vi "Autonomous Independent.vi"() -> ()   [LabVIEW 2019]
doc: "This VI is called when autonomous begins, and will automatically be terminated when autonomous ends. You can carry out timed or sensor driven robot movement independently without needing to return to the caller."
uses:
  <vilib>/Rock Robotics/WPI/Solenoid/WPI_SolenoidValue.ctl
  <vilib>/Rock Robotics/WPI/Utilities/WPI_GetSetVariantRefNum.vi
  <vilib>/Rock Robotics/Network Tables/NT Read String.vi
  <vilib>/Rock Robotics/Network Tables/NT Write Numeric Array.vi
  <vilib>/Rock Robotics/WPI/RobotDrive/WPI_RobotDriveArcadeDrive_Standard(NoSaturation).vi
  <vilib>/Rock Robotics/WPI/Solenoid/WPI_SolenoidSetEnum.vi
panel:
  in  "Polycord 3":dbl=-0.8 format="%#_13g"
  in  "Polycord 2":dbl=-0.8 format="%#_13g"
  in  "Angle 2":dbl
  in  "Speed 2":dbl
  in  "radius 2":dbl=20.0
  in  "angle 2":dbl=100.0
  in  "Inches Forward 2":dbl=26.0
  in  "Angle":dbl
  in  "Speed":dbl
  in  "radius":dbl=20.0
  in  "angle":dbl=100.0
  in  "Inches Forward":dbl=26.0
  # "Be sure to right-click and choose Data Operations>>Make Current Value default if you want to save the array values with the VI"
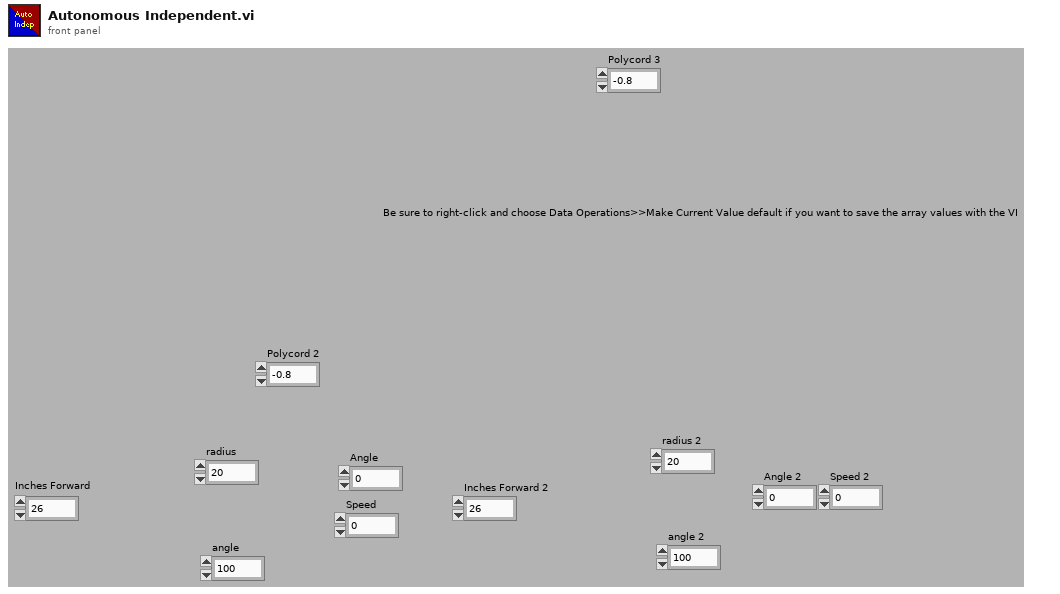
[diagram p1: front panel]
types:
  T1 = typedef "WPI_JoystickDevRef.ctl" = cluster{"Device":T2}
  T2 = typedef "WPI_JoystickDeviceEnum.ctl" = enum16{"USB 0", "USB 1", "USB 2", "USB 3", "USB 4", "USB 5"}
  T3 = typedef "WPI_SolenoidValue.ctl" = enum16{"Off", "On", "Forward", "Reverse"}
  T4 = typedef "WPI_RobotDriveDevRef.ctl" = cluster{"DevStatus":errorcluster, "Motors[]":T5[], "Square Inputs":bool, "Max Output":dbl}
  T5 = typedef "WPI_MotorControlDeviceRef.ctl" = cluster{"DeviceStatus":errorcluster, "Type":T6, "PWM":cluster{"PWM Channel":T7, "DeadBand":T8}, "CAN":cluster{"Device Number":u8, "SetOutput VI Ref":variant, "GetOutput VI Ref":variant, "Enable VI Ref":variant, "Disable VI Ref":variant, "Data":variant}, "Invert":bool, "DIO PWM":cluster{"PWM \"Enable\" Channel":T7, "DIOChannel":T9, "PWM Rate":dbl}}
  T6 = typedef "WPI_MotorControlType.ctl" = enum16{"PWM", "CAN", "DIO PWM"}
  T7 = typedef "FPGA_DIOPWMChannel.ctl" = enum8{"PWM 0", "PWM 1", "PWM 2", "PWM 3", "PWM 4", "PWM 5", "PWM 6", "PWM 7", "PWM 8", "PWM 9", "PWM MXP 0", "PWM MXP 1", "PWM MXP 2", "PWM MXP 3", "PWM MXP 4", "PWM MXP 5", "PWM MXP 6", "PWM MXP 7", "PWM MXP 8", "PWM MXP 9", "Invalid"}
  T8 = typedef "WPI_PWMDeadband.ctl" = cluster{"Name":string, "maxPositivePwm":i32, "minPositivePwm":i32, "centerPwm":i32, "maxNegativePwm":i32, "minNegativePwm":i32, "angularRange":u16}
  T9 = typedef "FPGA_DIOChannel.ctl" = enum8{"DIO 0", "DIO 1", "DIO 2", "DIO 3", "DIO 4", "DIO 5", "DIO 6", "DIO 7", "DIO 8", "DIO 9", "DIO MXP 0", "DIO MXP 1", "DIO MXP 2", "DIO MXP 3", "DIO MXP 4", "DIO MXP 5", "DIO MXP 6", "DIO MXP 7", "DIO MXP 8", "DIO MXP 9", "DIO MXP 10", "DIO MXP 11", "DIO MXP 12", "DIO MXP 13", "DIO MXP 14", "DIO MXP 15", "SPI Port CS1", "SPI Port CS2", "SPI Port CS3", "SPI Port MISO", "SPI Port MOSI", "Invalid"}
  T10 = typedef "WPI_SolenoidDevRef.ctl" = cluster{"DevStatus":errorcluster, "Pneumatics Control Module":u8, "Forward Solenoid Channel":T11, "Reverse Solenoid Channel":T11}
  T11 = typedef "WPI_SolenoidChannel.ctl" = enum8{"Solenoid 0", "Solenoid 1", "Solenoid 2", "Solenoid 3", "Solenoid 4", "Solenoid 5", "Solenoid 6", "Solenoid 7", "Invalid"}
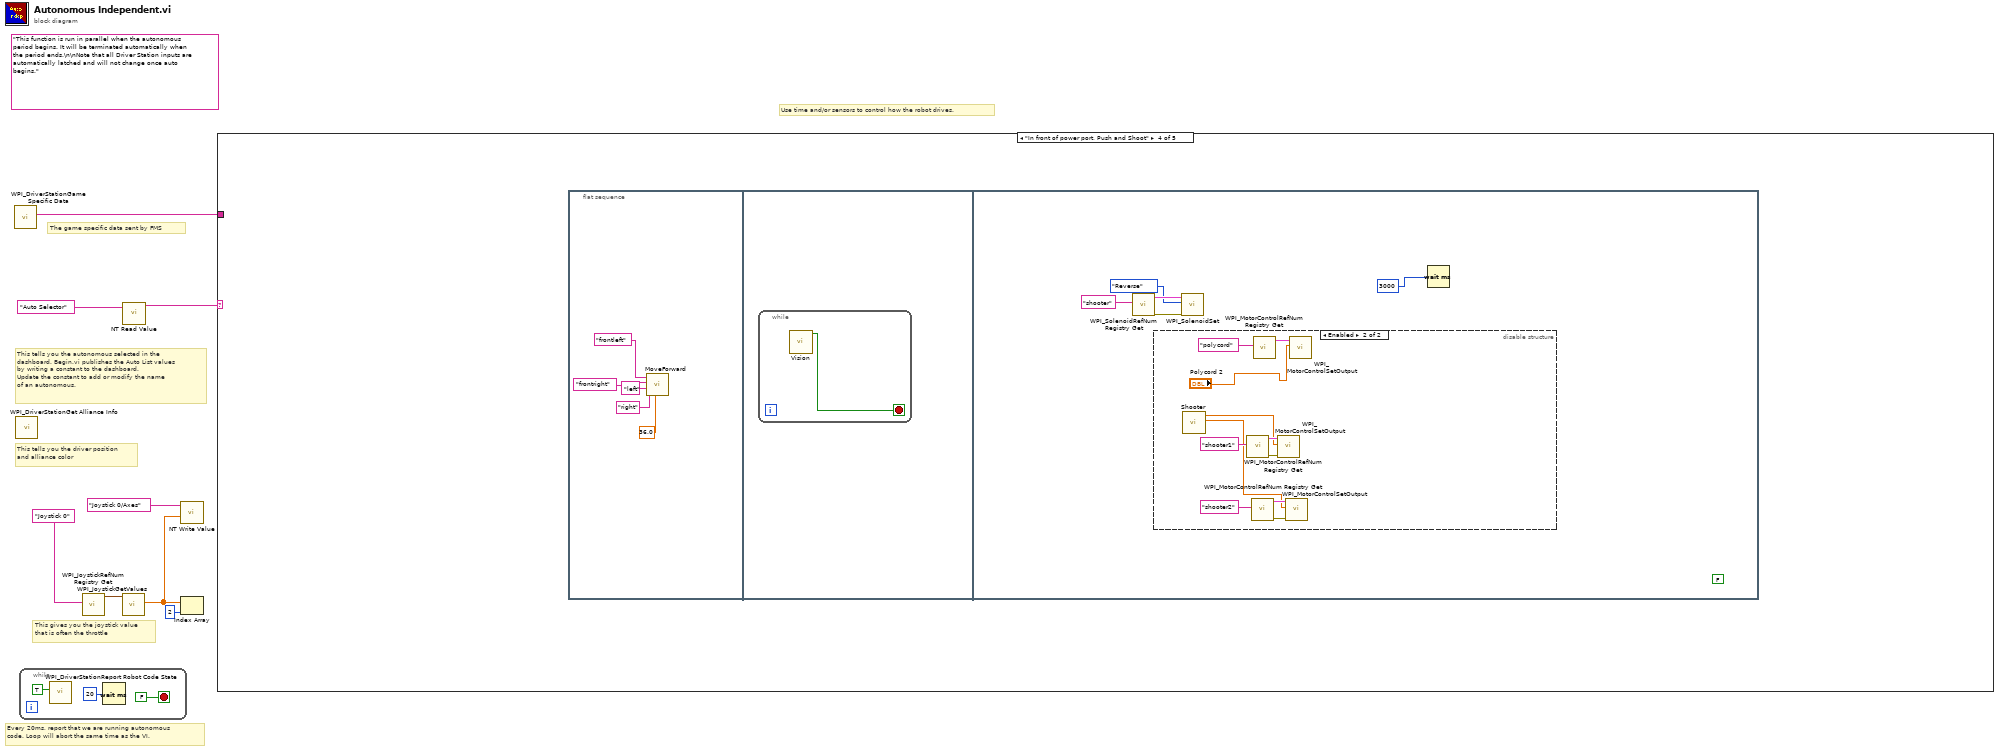
[diagram p0: block diagram]
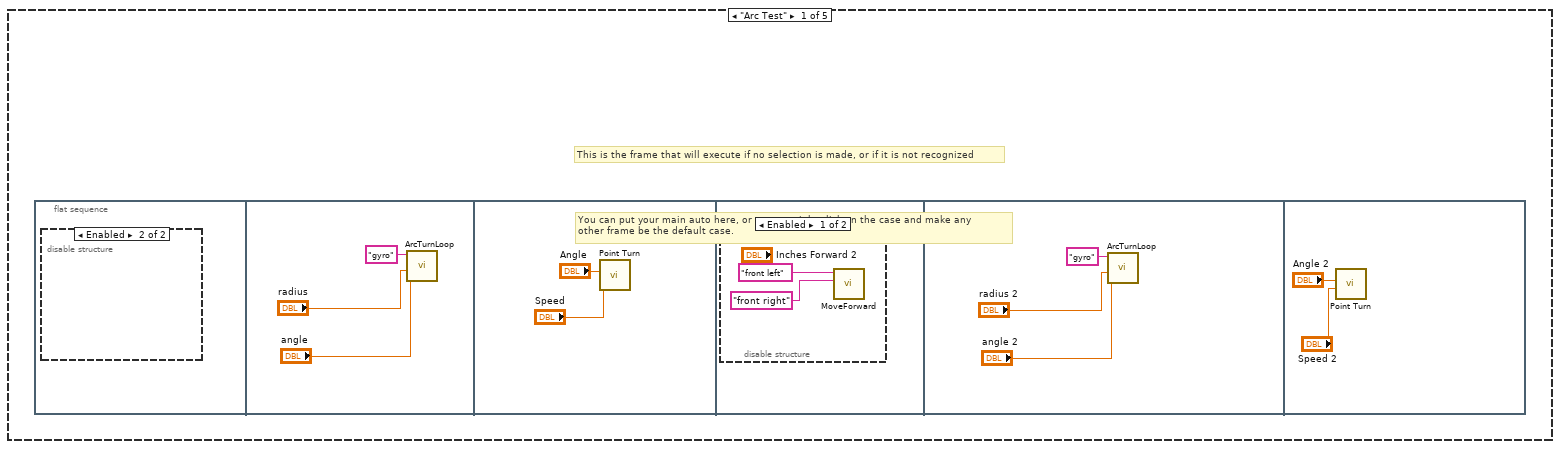
[diagram p2: hidden frame]
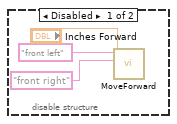
[diagram p3: hidden frame]
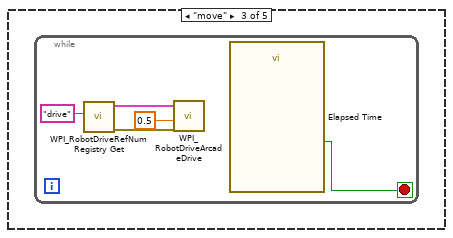
[diagram p6: hidden frame]
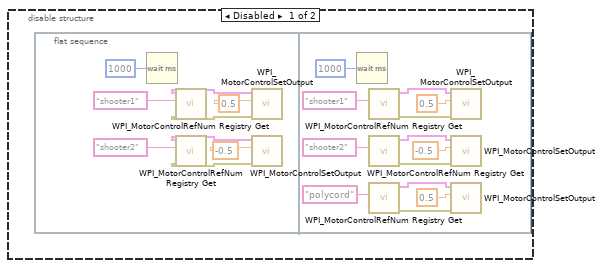
[diagram p7: hidden frame]
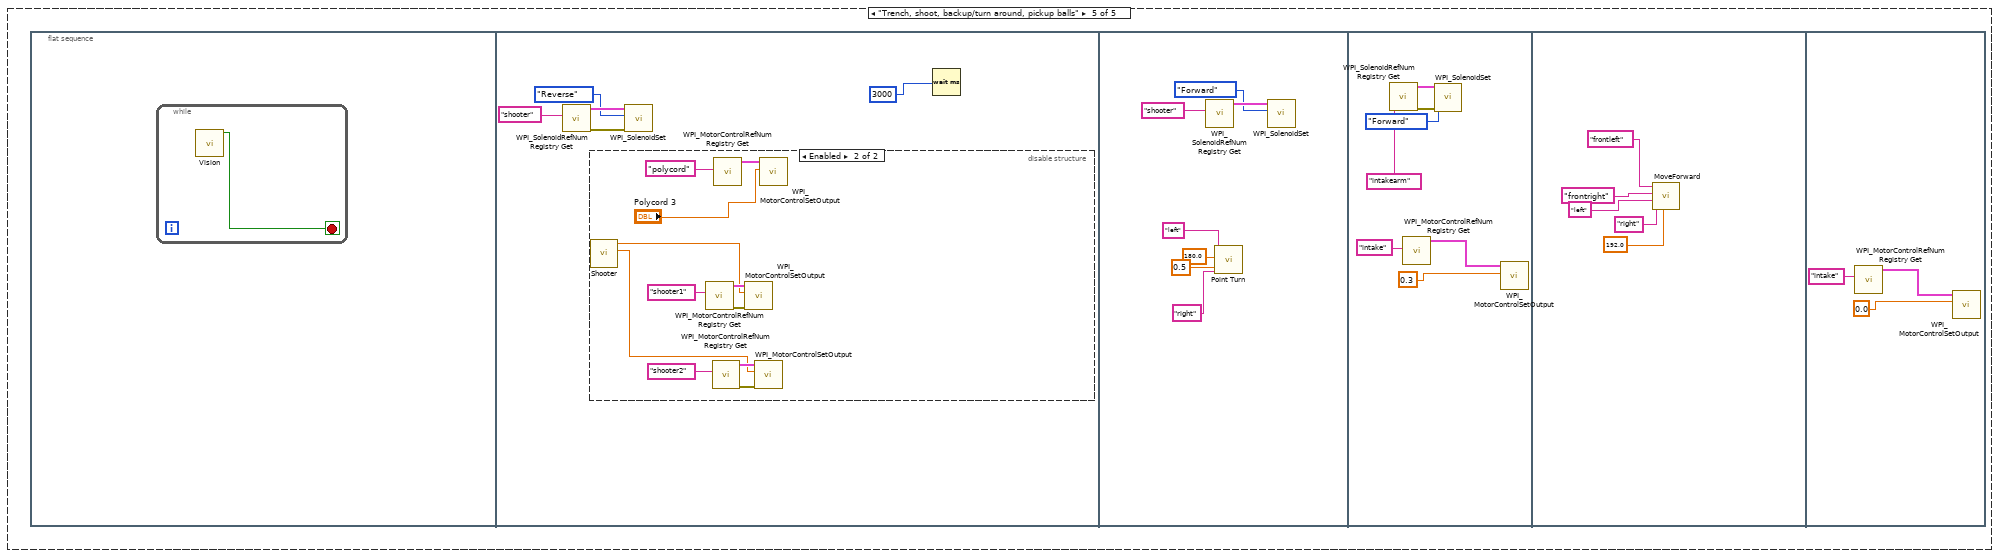
[diagram p8: hidden frame]
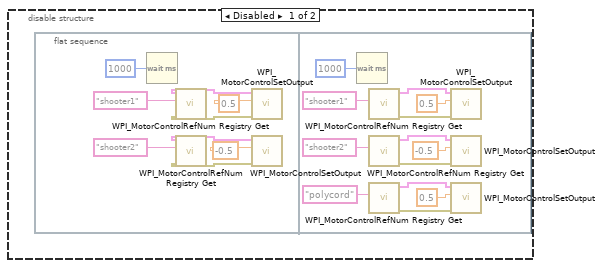
[diagram p9: hidden frame]
diagram:
  (unwired) "This function is run in parallel when the autonomous period begins. It will be terminated automatically when the period ends.\n\nNote that all Driver Station inputs are automatically latched and will not change once auto begins."
  # "The game specific data sent by FMS"
  # "This tells you the autonomous selected in the \ndashboard. Begin.vi publishes the Auto List values\nby writing a constant to the dashboard.\nUpdate the constant to add or modify the name\nof an autonomous."
  # "Every 20ms, report that we are running autonomous\ncode. Loop will abort the same time as the VI."
  # "This gives you the joystick value\nthat is often the throttle"
  # "Use time and/or sensors to control how the robot drives."
  # "This tells you the driver position\nand alliance color"
  n1 = call <vilib>:"WPI_DriverStationGame Specific Data.vi"() -> ("Game Specific Data"=w1:string)  [unwired: 11 in]
  n2 = call <vilib>:"WPI_DriverStationGet Alliance Info.vi"() -> ()  [unwired: 12 out]
  n3 = while {
    stop <- FALSE stop-if-true
    n4 = call <vilib>:"WPI_DriverStationReport Robot Code State.vi"("Autonomous"=TRUE) -> ()  [unwired: 10 in, 1 out]
    n5 = Wait (ms)(milliseconds to wait=u32 20) -> ()  [unwired: 1 out]
  }
  n6 = call <vilib>:"WPI_JoystickRefNum Registry Get.vi"("refnum name"="Joystick 0") -> ("JoystickDevRef"=w7:T1)  [unwired: 1 in, 9 out]
  n7 = call <vilib>:"WPI_JoystickGetValues.vi"("JoystickDevRef"=w7) -> ("Axes"=w3:dbl[])  [unwired: 6 in, 4 out]
  n8 = call-poly <vilib>:"NT Read Value.vi"("Name"="Auto Selector") -> ("String"=w4:string)  [unwired: 9 in, 1 out]
  n9 = call-poly <vilib>:"NT Write Value.vi"("Numeric Array"=w3, "Name"="Joystick 0/Axes") -> ()  [unwired: 9 in, 1 out]
  n10 = Index Array(array=w3, index=2) -> ()  [unwired: 1 out]
  n11 = case shown="\"In front of power port, Push and Shoot\"" w4 {
    tunnel: w1 -> [_ _ _ _ _]
    frame "Arc Test" {
      # "You can put your main auto here, or you can right-click on the case and make any\nother frame be the default case."
      # "This is the frame that will execute if no selection is made, or if it is not recognized"
      n12 = flat-sequence {
        frame #0 {
          n13 = disable-structure shown="Enabled" {
            frame Disabled {
              n14 = call "MoveForward.vi"("left motors"="Inches Forward", "right encoder"="front right" ("refnum name"), "left encoder"="front left" ("refnum name")) -> ()  [unwired: 9 in]
            }
            frame Enabled {
            }
          }
        }
        frame #1 {
          n15 = call "ArcTurnLoop.vi"("angle"="angle", "radius"="radius", "Gyro"="gyro") -> ()  [unwired: 9 in]
        }
        frame #2 {
          n16 = call "Point Turn.vi"("Speed"="Speed", "Angle"="Angle") -> ()  [unwired: 10 in]
        }
        frame #3 {
          n17 = disable-structure shown="Enabled" {
            frame Enabled {
              n18 = call "MoveForward.vi"("right encoder"="front right" ("refnum name"), "left encoder"="front left" ("refnum name")) -> ()  [unwired: 10 in]
            }
            frame Disabled {
            }
          }
        }
        frame #4 {
          n19 = call "ArcTurnLoop.vi"("angle"="angle 2", "radius"="radius 2", "Gyro"="gyro") -> ()  [unwired: 9 in]
        }
        frame #5 {
          n20 = call "Point Turn.vi"("Speed"="Speed 2", "Angle"="Angle 2") -> ()  [unwired: 10 in]
        }
      }
    }
    frame Default {
    }
    frame "move" {
      n21 = while {
        stop <- w27 stop-if-true
        n22 = call <vilib>:"WPI_RobotDriveRefNum Registry Get.vi"("refnum name"="drive") -> ("error out"=w29:errorcluster, "RobotDriveDevRef"=w30:T4)  [unwired: 9 in]
        n23 = call-poly <vilib>:"WPI_RobotDriveArcadeDrive.vi"("error in (no error)"=w29, "Y axis value"=0.5, "RobotDriveDevRef"=w30) -> ()  [unwired: 6 in, 3 out]
        n24 = call "Elapsed Time"() -> ("Time has Elapsed"=w27:bool)  [unwired: 12 in, 7 out]
      }
    }
    frame "In front of power port, Push and Shoot" {
      n25 = flat-sequence {
        frame #0 {
          n26 = call "MoveForward.vi"("Inches Forward"=36.0, "right motors"="right", "left motors"="left", "right encoder"="frontright" ("right motor controller"), "left encoder"="frontleft" ("left motor controller")) -> ()  [unwired: 7 in]
        }
        frame #1 {
          n27 = while {
            stop <- w37 stop-if-true
            n28 = call "Vision.vi"() -> ("Done?"=w37:bool)  [unwired: 11 in]
          }
        }
        frame #2 {
          (unwired) FALSE
          n29 = call <vilib>:"WPI_SolenoidRefNum Registry Get.vi"("refnum name"="shooter") -> ("error out"=w41:errorcluster, "SolenoidDevRef"=w40:T10)  [unwired: 9 in]
          n30 = disable-structure shown="Enabled" {
            frame Disabled {
              n31 = flat-sequence {
                frame #0 {
                  n32 = Wait (ms)(milliseconds to wait=u32 1000) -> ()  [unwired: 1 out]
                  n33 = call <vilib>:"WPI_MotorControlRefNum Registry Get.vi"("refnum name"="shooter1") -> ("error out"=w50:errorcluster, "MotorControlDevRef"=w49:T5)  [unwired: 9 in]
                  n34 = call <vilib>:"WPI_MotorControlRefNum Registry Get.vi"("refnum name"="shooter2") -> ("error out"=w47:errorcluster, "MotorControlDevRef"=w46:T5)  [unwired: 9 in]
                  n35 = call <vilib>:"WPI_MotorControlSetOutput.vi"("error in (no error)"=w50, "Output"=0.5, "MotorControlDevRef"=w49) -> ()  [unwired: 6 in, 3 out]
                  n36 = call <vilib>:"WPI_MotorControlSetOutput.vi"("error in (no error)"=w47, "Output"=-0.5, "MotorControlDevRef"=w46) -> ()  [unwired: 6 in, 3 out]
                }
                frame #1 {
                  n37 = Wait (ms)(milliseconds to wait=u32 1000) -> ()  [unwired: 1 out]
                  n38 = call <vilib>:"WPI_MotorControlRefNum Registry Get.vi"("refnum name"="shooter1") -> ("error out"=w63:errorcluster, "MotorControlDevRef"=w62:T5)  [unwired: 9 in]
                  n39 = call <vilib>:"WPI_MotorControlRefNum Registry Get.vi"("refnum name"="shooter2") -> ("error out"=w59:errorcluster, "MotorControlDevRef"=w58:T5)  [unwired: 9 in]
                  n40 = call <vilib>:"WPI_MotorControlRefNum Registry Get.vi"("refnum name"="polycord") -> ("error out"=w55:errorcluster, "MotorControlDevRef"=w54:T5)  [unwired: 9 in]
                  n41 = call <vilib>:"WPI_MotorControlSetOutput.vi"("error in (no error)"=w63, "Output"=0.5, "MotorControlDevRef"=w62) -> ()  [unwired: 6 in, 3 out]
                  n42 = call <vilib>:"WPI_MotorControlSetOutput.vi"("error in (no error)"=w59, "Output"=-0.5, "MotorControlDevRef"=w58) -> ()  [unwired: 6 in, 3 out]
                  n43 = call <vilib>:"WPI_MotorControlSetOutput.vi"("error in (no error)"=w55, "Output"=0.5, "MotorControlDevRef"=w54) -> ()  [unwired: 6 in, 3 out]
                }
              }
            }
            frame Enabled {
              n44 = call "Shooter.vi"() -> ("Bottom"=w66:dbl, "Top"=w65:dbl)  [unwired: 10 in]
              n45 = call <vilib>:"WPI_MotorControlRefNum Registry Get.vi"("refnum name"="shooter1") -> ("error out"=w74:errorcluster, "MotorControlDevRef"=w73:T5)  [unwired: 9 in]
              n46 = call <vilib>:"WPI_MotorControlRefNum Registry Get.vi"("refnum name"="shooter2") -> ("error out"=w71:errorcluster, "MotorControlDevRef"=w70:T5)  [unwired: 9 in]
              n47 = call <vilib>:"WPI_MotorControlRefNum Registry Get.vi"("refnum name"="polycord") -> ("MotorControlDevRef"=w68:T5)  [unwired: 9 in, 1 out]
              n48 = call <vilib>:"WPI_MotorControlSetOutput.vi"("error in (no error)"=w74, "Output"=w65, "MotorControlDevRef"=w73) -> ()  [unwired: 6 in, 3 out]
              n49 = call <vilib>:"WPI_MotorControlSetOutput.vi"("error in (no error)"=w71, "Output"=w66, "MotorControlDevRef"=w70) -> ()  [unwired: 6 in, 3 out]
              n50 = call <vilib>:"WPI_MotorControlSetOutput.vi"("Output"="Polycord 2", "MotorControlDevRef"=w68) -> ()  [unwired: 7 in, 3 out]
            }
          }
          n51 = call-poly <vilib>:"WPI_SolenoidSet.vi"("error in (no error)"=w41, "Value"=WPI_SolenoidValue."Reverse", "SolenoidDevRef"=w40) -> ()  [unwired: 7 in, 2 out]
          n52 = Wait (ms)(milliseconds to wait=u32 3000) -> ()  [unwired: 1 out]
        }
      }
    }
    frame "Trench, shoot, backup/turn around, pickup balls" {
      n53 = flat-sequence {
        frame #0 {
          n54 = while {
            stop <- w76 stop-if-true
            n55 = call "Vision.vi"() -> ("Done?"=w76:bool)  [unwired: 11 in]
          }
        }
        frame #1 {
          n56 = call <vilib>:"WPI_SolenoidRefNum Registry Get.vi"("refnum name"="shooter") -> ("error out"=w80:errorcluster, "SolenoidDevRef"=w81:T10)  [unwired: 9 in]
          n57 = disable-structure shown="Enabled" {
            frame Disabled {
              n58 = flat-sequence {
                frame #0 {
                  n59 = Wait (ms)(milliseconds to wait=u32 1000) -> ()  [unwired: 1 out]
                  n60 = call <vilib>:"WPI_MotorControlRefNum Registry Get.vi"("refnum name"="shooter1") -> ("error out"=w89:errorcluster, "MotorControlDevRef"=w88:T5)  [unwired: 9 in]
                  n61 = call <vilib>:"WPI_MotorControlRefNum Registry Get.vi"("refnum name"="shooter2") -> ("error out"=w86:errorcluster, "MotorControlDevRef"=w85:T5)  [unwired: 9 in]
                  n62 = call <vilib>:"WPI_MotorControlSetOutput.vi"("error in (no error)"=w89, "Output"=0.5, "MotorControlDevRef"=w88) -> ()  [unwired: 6 in, 3 out]
                  n63 = call <vilib>:"WPI_MotorControlSetOutput.vi"("error in (no error)"=w86, "Output"=-0.5, "MotorControlDevRef"=w85) -> ()  [unwired: 6 in, 3 out]
                }
                frame #1 {
                  n64 = Wait (ms)(milliseconds to wait=u32 1000) -> ()  [unwired: 1 out]
                  n65 = call <vilib>:"WPI_MotorControlRefNum Registry Get.vi"("refnum name"="shooter1") -> ("error out"=w102:errorcluster, "MotorControlDevRef"=w101:T5)  [unwired: 9 in]
                  n66 = call <vilib>:"WPI_MotorControlRefNum Registry Get.vi"("refnum name"="shooter2") -> ("error out"=w98:errorcluster, "MotorControlDevRef"=w97:T5)  [unwired: 9 in]
                  n67 = call <vilib>:"WPI_MotorControlRefNum Registry Get.vi"("refnum name"="polycord") -> ("error out"=w94:errorcluster, "MotorControlDevRef"=w93:T5)  [unwired: 9 in]
                  n68 = call <vilib>:"WPI_MotorControlSetOutput.vi"("error in (no error)"=w102, "Output"=0.5, "MotorControlDevRef"=w101) -> ()  [unwired: 6 in, 3 out]
                  n69 = call <vilib>:"WPI_MotorControlSetOutput.vi"("error in (no error)"=w98, "Output"=-0.5, "MotorControlDevRef"=w97) -> ()  [unwired: 6 in, 3 out]
                  n70 = call <vilib>:"WPI_MotorControlSetOutput.vi"("error in (no error)"=w94, "Output"=0.5, "MotorControlDevRef"=w93) -> ()  [unwired: 6 in, 3 out]
                }
              }
            }
            frame Enabled {
              n71 = call "Shooter.vi"() -> ("Bottom"=w104:dbl, "Top"=w105:dbl)  [unwired: 10 in]
              n72 = call <vilib>:"WPI_MotorControlRefNum Registry Get.vi"("refnum name"="shooter1") -> ("error out"=w113:errorcluster, "MotorControlDevRef"=w112:T5)  [unwired: 9 in]
              n73 = call <vilib>:"WPI_MotorControlRefNum Registry Get.vi"("refnum name"="shooter2") -> ("error out"=w110:errorcluster, "MotorControlDevRef"=w109:T5)  [unwired: 9 in]
              n74 = call <vilib>:"WPI_MotorControlRefNum Registry Get.vi"("refnum name"="polycord") -> ("MotorControlDevRef"=w107:T5)  [unwired: 9 in, 1 out]
              n75 = call <vilib>:"WPI_MotorControlSetOutput.vi"("error in (no error)"=w113, "Output"=w105, "MotorControlDevRef"=w112) -> ()  [unwired: 6 in, 3 out]
              n76 = call <vilib>:"WPI_MotorControlSetOutput.vi"("error in (no error)"=w110, "Output"=w104, "MotorControlDevRef"=w109) -> ()  [unwired: 6 in, 3 out]
              n77 = call <vilib>:"WPI_MotorControlSetOutput.vi"("Output"="Polycord 3", "MotorControlDevRef"=w107) -> ()  [unwired: 7 in, 3 out]
            }
          }
          n78 = call-poly <vilib>:"WPI_SolenoidSet.vi"("error in (no error)"=w80, "Value"=WPI_SolenoidValue."Reverse", "SolenoidDevRef"=w81) -> ()  [unwired: 7 in, 2 out]
          n79 = Wait (ms)(milliseconds to wait=u32 3000) -> ()  [unwired: 1 out]
        }
        frame #2 {
          n80 = call <vilib>:"WPI_SolenoidRefNum Registry Get.vi"("refnum name"="shooter") -> ("SolenoidDevRef"=w121:T10)  [unwired: 9 in, 1 out]
          n81 = call "Point Turn.vi"("right motors"="right" ("right"), "Speed"=0.5, "Angle"=180.0, "left motors"="left" ("left")) -> ()  [unwired: 8 in]
          n82 = call-poly <vilib>:"WPI_SolenoidSet.vi"("Value"=WPI_SolenoidValue."Forward", "SolenoidDevRef"=w121) -> ()  [unwired: 8 in, 2 out]
        }
        frame #3 {
          n83 = call <vilib>:"WPI_SolenoidRefNum Registry Get.vi"("refnum name"="intakearm") -> ("error out"=w125:errorcluster, "SolenoidDevRef"=w124:T10)  [unwired: 9 in]
          n84 = call <vilib>:"WPI_MotorControlRefNum Registry Get.vi"("refnum name"="intake") -> ("MotorControlDevRef"=w128:T5)  [unwired: 9 in, 1 out]
          n85 = call-poly <vilib>:"WPI_SolenoidSet.vi"("error in (no error)"=w125, "Value"=WPI_SolenoidValue."Forward", "SolenoidDevRef"=w124) -> ()  [unwired: 7 in, 2 out]
          n86 = call <vilib>:"WPI_MotorControlSetOutput.vi"("Output"=0.3, "MotorControlDevRef"=w128) -> ()  [unwired: 7 in, 3 out]
        }
        frame #4 {
          n87 = call "MoveForward.vi"("Inches Forward"=192.0, "right motors"="right", "left motors"="left", "right encoder"="frontright" ("right motor controller"), "left encoder"="frontleft" ("left motor controller")) -> ()  [unwired: 7 in]
        }
        frame #5 {
          n88 = call <vilib>:"WPI_MotorControlRefNum Registry Get.vi"("refnum name"="intake") -> ("MotorControlDevRef"=w136:T5)  [unwired: 9 in, 1 out]
          n89 = call <vilib>:"WPI_MotorControlSetOutput.vi"("Output"=0.0, "MotorControlDevRef"=w136) -> ()  [unwired: 7 in, 3 out]
        }
      }
    }
  }
